vi "Clear RTDriver VIs File Paths.vi"(8 "error in":errorcluster, 11 "Item Ref in":u64 format="%.0x") -> (0 "error out":errorcluster, 3 "Item Ref out":u64 format="%.0x")   [LabVIEW 2026, in "SystemMonitor Configuration.lvlib"]
uses:
  SystemMonitor Configuration.lvlib
  NationalInstruments.VeriStand.SystemStorage
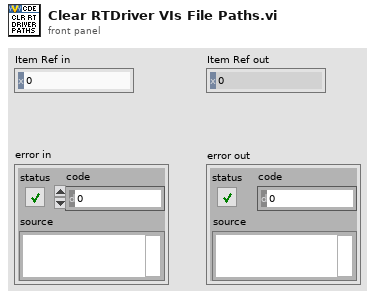
[diagram p1: front panel]
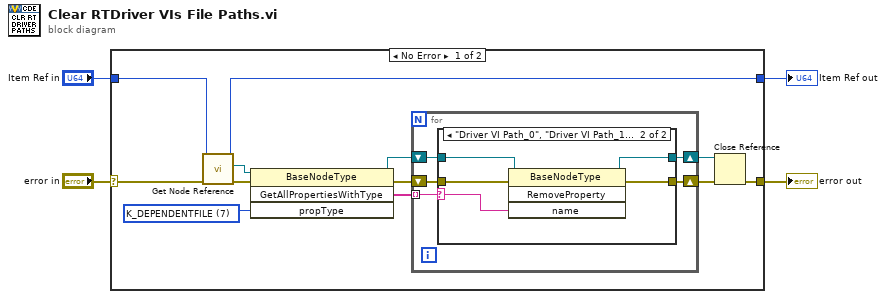
[diagram p0: block diagram]
diagram:
  n1 = case shown="No Error" "error in" {
    selector: "error in" -> [w15 w30]
    tunnel: "Item Ref in" -> [w14 w29]
    tunnel: [w13 w29] -> w2
    tunnel: [w16 w30] -> w1
    frame No Error {
      w11 = 7 items=["K_STRING", "K_BOOL", "K_I32", "K_U32", "K_DOUBLE", "K_U64", "K_VARIANT", "K_DEPENDENTFILE", "K_DEPENDENTNODE", "K_DATASOURCENODE", "K_U16", "K_DBLARR", "K_U32ARR", "K_I32ARR", "K_STRINGARR", "K_DICTIONARY", "K_DICTIONARYARR", "K_BINARYSTRING", "K_I16", "K_I64", "K_BOOLARR", "K_U64ARR", "K_U16ARR", "K_I64ARR", "K_I16ARR"] ("propType")
      n2 = call "Get Node Reference.vi"("error in"=w15, "Item Ref in"=w14) -> ("error out"=w6:errorcluster, "Base Node Type"=w5:refnum<k24>, "Item Ref out"=w13:u64)  [unwired: 6 in, 1 out]
      n3 = invoke class="BaseNodeType" method="GetAllPropertiesWithType"(reference=w5, error in=w6, "propType"=w11) -> (reference out=w10:refnum<k24>, error out=w12:errorcluster, "GetAllPropertiesWithType"=w9:string[])  [unwired: 1 in, 1 out]
      n4 = for {
        tunnel: w9 -> [w17] mode=indexing
        shift-right: [w19] -> w8
        shift-left: w12 -> [w20]
        shift-right: [w18] -> w7
        shift-left: w10 -> [w21]
        n5 = case shown="\"Driver VI Path_0\", \"Driver VI Path_1\", \"Driver VI Path_2\", \"Driver VI Path_3\", \"Driver VI Path_4\"" w17 {
          selector: w17 -> [_ w24]
          tunnel: w21 -> [w23 w28]
          tunnel: w20 -> [w22 w27]
          tunnel: [w22 w26] -> w19
          tunnel: [w23 w25] -> w18
          frame "None", Default {
          }
          frame "Driver VI Path_0", "Driver VI Path_1", "Driver VI Path_2", "Driver VI Path_3", "Driver VI Path_4" {
            n6 = invoke class="BaseNodeType" method="RemoveProperty"(reference=w28, error in=w27, "name"=w24) -> (reference out=w25:refnum<k24>, error out=w26:errorcluster)  [unwired: 1 in, 2 out]
          }
        }
      }
      n7 = Close Reference(reference=w7, error in (no error)=w8) -> (error out=w16:errorcluster)
    }
    frame Error {
    }
  }
  "Item Ref out" <- w2
  "error out" <- w1
